vi "Simulation of Tomography.vi"() -> ()   [LabVIEW 2023]
doc: "Simulates the analog reconstruction of the interior of a nontransparent body. This kind of tomography uses X-rays. Given 3 flaws in the interior of a nontransparent body and based on a collection of single images, the analog reconstruction is realized."
panel:
  out "results":dbl[][](graph)
  out "current scan":dbl[][](graph)
  in  "number of takes":i32=25 min=10 max=100 step=1
  out "real situation with 3 flaws":cluster{dbl[], dbl[]}[](graph)
  # "Overview: Simulates the analog reconstruction of the interior of a nontransparent body.\nInstructions: \nRun the VI. Note that the 3 flaws in the interior of the nontransparent body are reconstructed in the results."
  # "Note: This example does not use any of the Mathematics VIs. All of the calculations are performed with simple numeric functions and Formula Nodes."
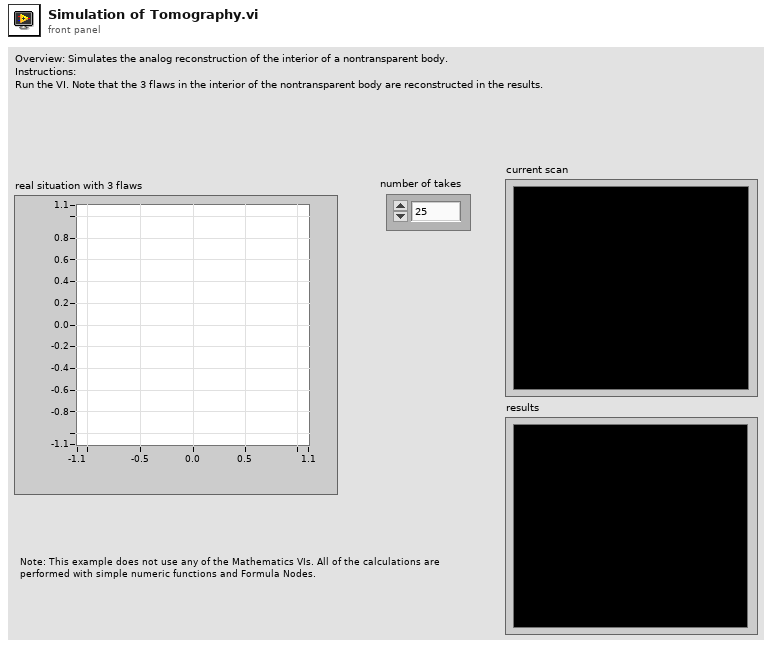
[diagram p1: front panel]
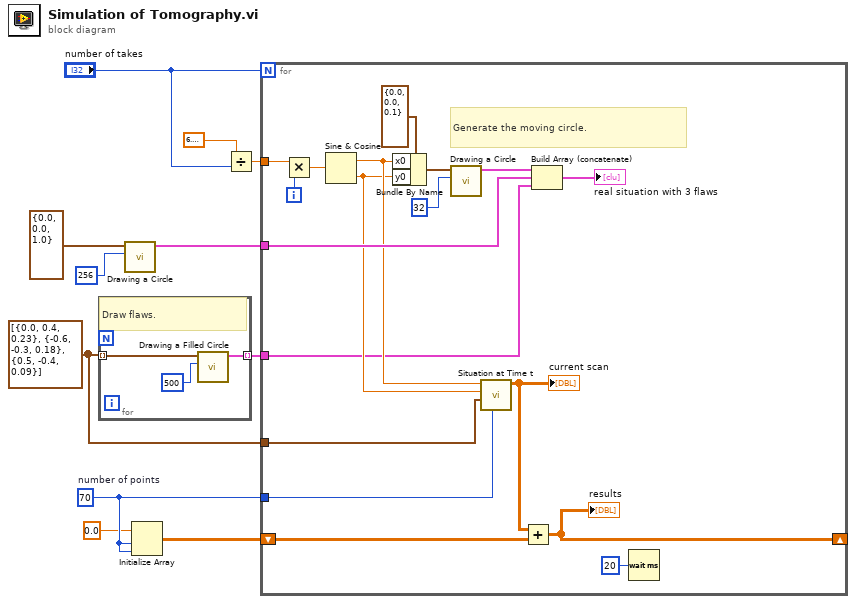
[diagram p0: block diagram]
diagram:
  w3 = cluster{"x0":dbl, "y0":dbl, "r":dbl}[] [{"x0"=0.0, "y0"=0.4, "r"=0.23}, {"x0"=-0.6, "y0"=-0.3, "r"=0.18}, {"x0"=0.5, "y0"=-0.4, "r"=0.09}] ("appended array")
  w7 = 70  # number of points
  n1 = for {
    tunnel: w3 -> [w14] mode=indexing
    tunnel: [w13] -> w4 mode=indexing
    # "Draw flaws."
    n2 = call "Drawing a Filled Circle.vi"("number of points"=500, "circle"=w14) -> ("circle graph"=w13:cluster{"x":dbl[], "y":dbl[]})  [unwired: 9 in]
  }
  n3 = call "Drawing a Circle.vi"("number of points"=256, "circle"=cluster{"x0":dbl, "y0":dbl, "r":dbl} {"x0"=0.0, "y0"=0.0, "r"=1.0}) -> ("circle graph"=w8:cluster{"x":dbl[], "y":dbl[]})  [unwired: 9 in]
  n4 = Initialize Array(0.0, w7, w7) -> (w6:dbl[][])
  n5 = Divide(x=6.283185307179586, y="number of takes") -> (x/y=w9:dbl)
  n6 = for {
    N: "number of takes" -> [_]
    tunnel: w9 -> [w31]
    tunnel: w8 -> [w26]
    tunnel: w7 -> [w25]
    shift-right: [w15] -> _
    shift-left: w6 -> [w23]
    tunnel: w3 -> [w19]
    tunnel: w4 -> [w16]
    i -> [w32]
    # "Generate the moving circle."
    n7 = Multiply(x=w31, y=w32) -> (x*y=w30:dbl)
    n8 = Sine & Cosine(0:w30) -> (1:w18:dbl, 2:w17:dbl)
    n9 = Bundle By Name(cluster=cluster{"x0":dbl, "y0":dbl, "r":dbl} {"x0"=0.0, "y0"=0.0, "r"=0.1} ("circle"), "x0"=w18, "y0"=w17) -> (w20:cluster{"x0":dbl, "y0":dbl, "r":dbl})
    n10 = call "Drawing a Circle.vi"("number of points"=32, "circle"=w20) -> ("circle graph"=w27:cluster{"x":dbl[], "y":dbl[]})  [unwired: 9 in]
    n11 = call "Situation at Time t.vi"("number of points"=w25, "flaws (circles)"=w19, "y source"=w17, "x source"=w18) -> ("tomography array"=w24:dbl[][])  [unwired: 7 in]
    "current scan" <- w24
    n12 = Add(x=w24, y=w23) -> (x+y=w15:dbl[][])
    "results" <- w15
    n13 = Build Array (concatenate)(w27, w26, w16) -> (→"real situation with 3 flaws":cluster{"x":dbl[], "y":dbl[]}[])
    n14 = Wait (ms)(milliseconds to wait=u32 20) -> ()  [unwired: 1 out]
  }
